vi "Initialize.vi"(0 "RS NRPx Power Meter in":refnum<class "Power Meter.lvclass">, 11 "error in":errorcluster) -> (4 "RS NRPx Power Meter out":refnum<class "Power Meter.lvclass">, 15 "error out":errorcluster)   [LabVIEW 2023, in "RS NRPx Power Meter.lvlib" / "Power Meter.lvclass"]
uses:
  Power Meter.lvclass
  Instruments/Power Meter/Power Meter Base/Power Meter Base.lvclass/Power Meter Base.ctl
  Power Meter.lvclass/Power Meter.ctl
  Instruments/Power Meter/Power Meter Base/Properties/Read Active Instrument Info.vi
  <instrlib>/Rohde&Schwarz Power Meter/Rohde&Schwarz Power Meter.lvlib
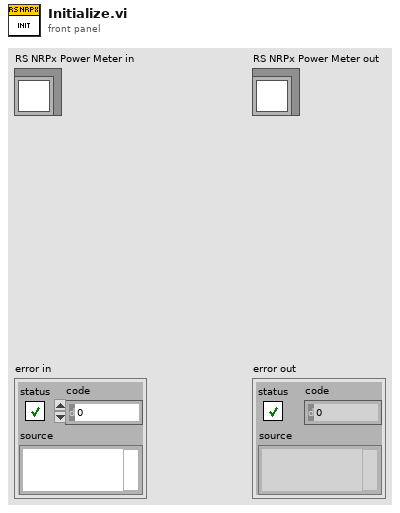
[diagram p1: front panel]
types:
  T1 = typedef "RFFixtureCharact.Instruments.lvlib/Power Meter Base.lvclass/Instrument Info.ctl" = cluster{"User Alias":string, "Resource Name":string, "Product Name":string, "Vendor Name":string}
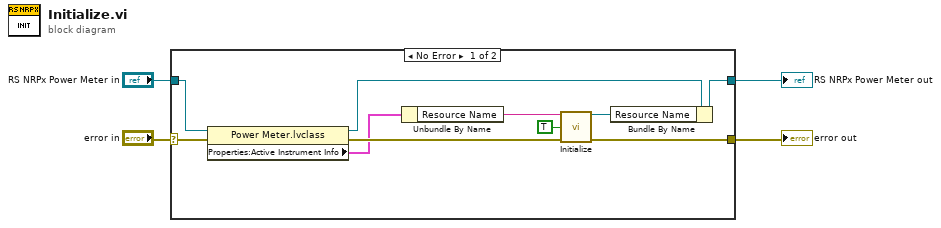
[diagram p0: block diagram]
diagram:
  n1 = case shown="No Error" "error in" {
    selector: "error in" -> [w12 w16]
    tunnel: [w13 w16] -> w1
    tunnel: "RS NRPx Power Meter in" -> [w9 w15]
    tunnel: [w7 w15] -> w3
    frame No Error {
      n2 = property class="Power Meter.lvclass"(reference=w9, error in=w12) -> (reference out=w8:refnum<class "Power Meter.lvclass">, error out=w11:errorcluster, "Properties:Active Instrument Info"=w10:T1)
      n3 = Unbundle By Name(w10) -> ("Resource Name"=w6:string)
      n4 = call <instrlib>:"Initialize.vi"("VISA resource name"=w6, "Reset (T: Reset)"=TRUE ("reset device"), "error in (no error)"=w11) -> ("VISA resource name out"=w5:refnum<visa-resource-name>, "error out"=w13:errorcluster)  [unwired: 11 in]
      n5 = Bundle By Name(cluster=w8, "Resource Name"=w5) -> (w7:refnum<class "Power Meter.lvclass">)
    }
    frame Error {
    }
  }
  "error out" <- w1
  "RS NRPx Power Meter out" <- w3
